vi "Delete.vi"(8 "error in (no error)":errorcluster, 10 "Name":string, 11 "FSM.Annotation in":refnum<class "FSM.Annotation.lvclass">) -> (0 "error out":errorcluster, 2 "Changed?":bool, 3 "FSM.Annotation out":refnum<class "FSM.Annotation.lvclass">)   [LabVIEW 2015, in "FSM.Annotation.lvclass"]
uses:
  FSM.Annotation.lvclass
  FSM.Annotation.lvclass/FSM.Annotation.ctl
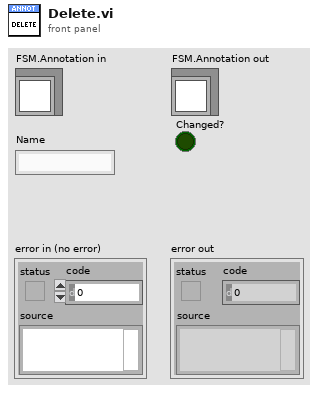
[diagram p1: front panel]
types:
  T1 = cluster{"Name":string, "Style":enum16{"Plain", "On", "Off", "On-Off"}}[]
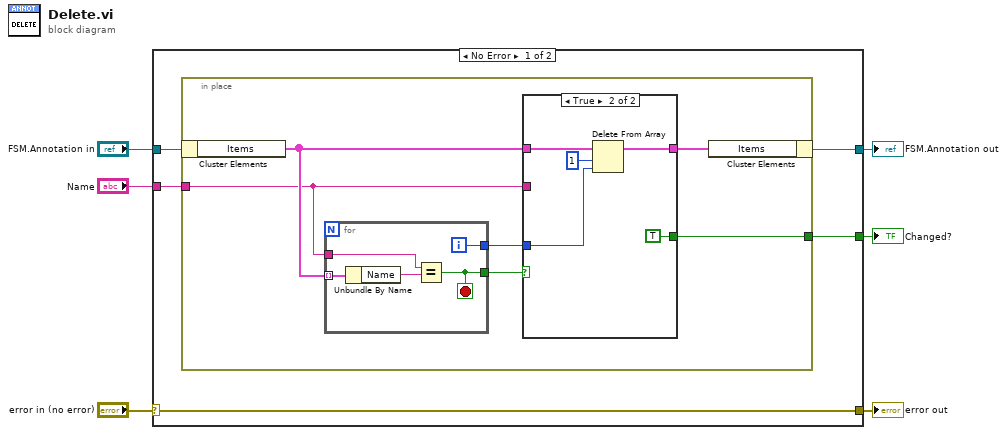
[diagram p0: block diagram]
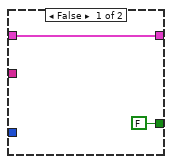
[diagram p2: hidden frame]
diagram:
  n1 = case shown="No Error" "error in (no error)" {
    selector: "error in (no error)" -> [w11 w31]
    tunnel: [w11 w31] -> w5
    tunnel: [w9 w30] -> w3
    tunnel: "FSM.Annotation in" -> [w10 w30]
    tunnel: "Name" -> [w8 _]
    tunnel: [w7 _] -> w1
    frame No Error {
      n2 = in-place {
        in-place-border: w8 -> [w14]
        in-place-border: [w12] -> w7
        n3 = in-place-cluster #1(w10) -> ("Items"=w15:T1)
        n4 = for {
          tunnel: w15 -> [w27] mode=indexing
          tunnel: w14 -> [w28]
          tunnel: [w26] -> w16
          tunnel: [w25] -> w17
          i -> [w25]
          stop <- w26 stop-if-true
          n5 = Unbundle By Name(w27) -> ("Name"=w29:string)
          n6 = Equal?(x=w28, y=w29) -> (x = y?=w26:bool)
        }
        n7 = case shown="True" w16 {
          tunnel: w15 -> [w19 w23]
          tunnel: w17 -> [_ w21]
          tunnel: [w19 w20] -> w13
          tunnel: w14 -> [_ _]
          tunnel: [FALSE TRUE] -> w12
          frame False {
          }
          frame True {
            n8 = Delete From Array(array=w23, length=1, index=w21) -> (array with subset deleted=w20:T1)  [unwired: 1 out]
          }
        }
        n9 = in-place-cluster #1("Items"=w13) -> (w9:refnum<class "FSM.Annotation.lvclass">)
      }
    }
    frame Error {
    }
  }
  "error out" <- w5
  "FSM.Annotation out" <- w3
  "Changed?" <- w1
